vi "Part2-6.vi"() -> ()   [LabVIEW 2016]
uses:
  <vilib>/sound2/lvsound2.llb/Sound Data Format.ctl
  <vilib>/sound2/lvsound2.llb/Sound File Info (path).vi
panel:
  in  "output":path
  out "output":waveform(dbl)(graph)
  out "sound format":T1={"sample rate (S/s)"=22050.0, "number of channels"=2, "bits per sample"=16}
  out "1/x":dbl
  out "dt":dbl
  out "Input":waveform(dbl)(graph)
  in  "input":path
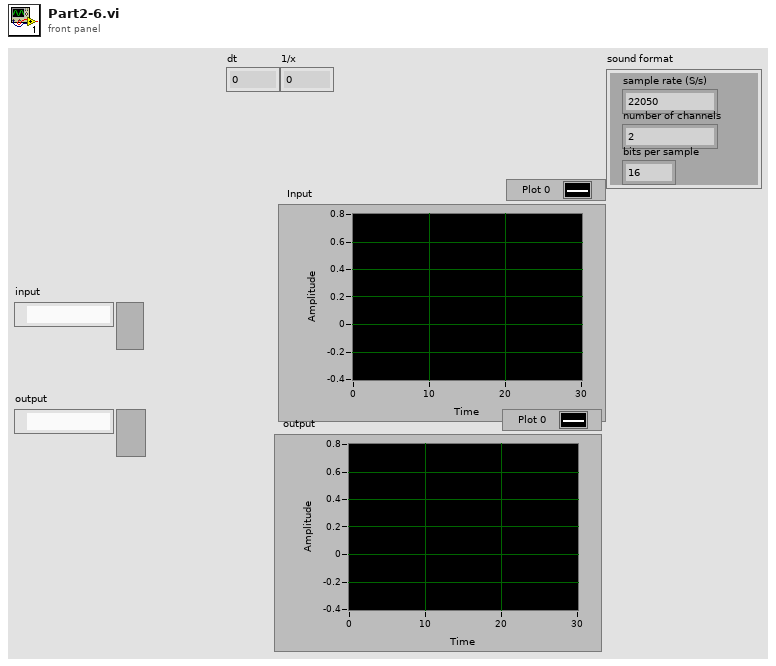
[diagram p1: front panel]
types:
  T1 = typedef "Sound Data Format.ctl" = cluster{"sample rate (S/s)":dbl, "number of channels":i32, "bits per sample":i32}
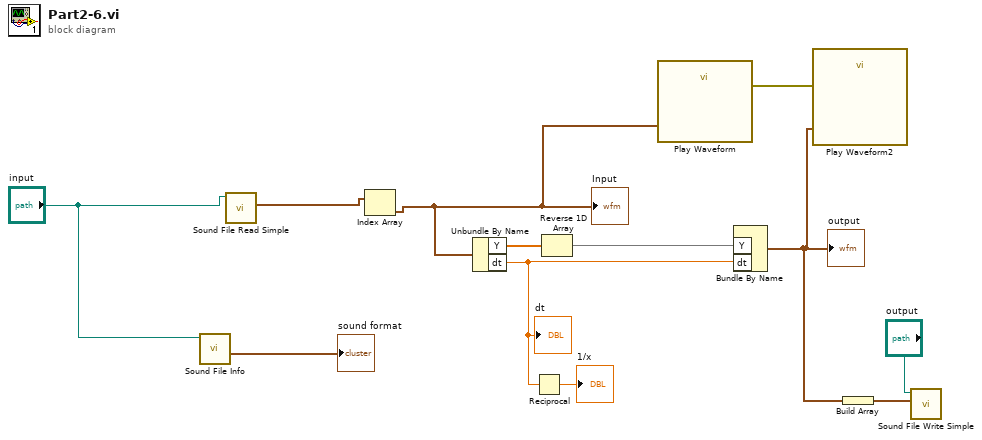
[diagram p0: block diagram]
diagram:
  n1 = call-poly <vilib>:"Sound File Info.vi"("path"="input") -> ("sound format"=→"sound format":T1)  [unwired: 7 in, 3 out]
  n2 = call <vilib>:"Sound File Read Simple.vi"("path"="input") -> ("data"=w12:waveform(dbl)[])  [unwired: 7 in, 3 out]
  n3 = Index Array(array=w12) -> (element=w5:waveform(dbl))  [unwired: 1 in]
  "Input" <- w5
  n4 = Unbundle By Name(w5) -> ("Y"=w11:dbl[], "dt"=w6:dbl)
  "dt" <- w6
  n5 = Reciprocal(x=w6) -> (1/x=→"1/x":dbl)
  n6 = Reverse 1D Array(array=w11) -> (reversed array=w7:dbl[])
  n7 = call "Play Waveform"("Data"=w5) -> ("error out"=w4:errorcluster)  [unwired: 18 in]
  n8 = Bundle By Name("Y"=w7, "dt"=w6) -> (w3:waveform(dbl))  [unwired: 1 in]
  "output" <- w3
  n9 = call "Play Waveform2"("Data"=w3, "error in"=w4) -> ()  [unwired: 17 in, 1 out]
  n10 = Build Array(w3) -> (w2:waveform(dbl)[])
  n11 = call <vilib>:"Sound File Write Simple.vi"("data"=w2, "path"="output") -> ()  [unwired: 8 in, 2 out]
